vi "ecg_ncs_v7.vi"() -> ()   [LabVIEW 2016]
uses:
  <instrlib>/niUSRP/niUSRP Timestamp.ctl
  C:/Program Files/National Instruments/LabVIEW 2016/examples/Instrument IO/Serial/support/Serial - Settings.ctl
  State.ctl
  <vilib>/Instr/_visa.llb/VISA Configure Serial Port (Instr).vi
  <instrlib>/niUSRP/niUSRP Fetch Rx Data (2D CDB).vi
  <instrlib>/niUSRP/niUSRP Write Tx Data (2D CDB).vi
panel:
  in  "Tab Control 3":enum32{"ECG Sample", "ECG"}(tab)
  out "?":i32(graph)
  out "?":i16(graph)
  in  "maxWrite":i32=2000
  out "size(s) 2":i32
  out "size(s)":i32
  in  "File Name 2":string="Test"
  in  "Path 2":path=path "D:/Research/SummerFall17Spring18/CnC/NCS/EcgNcsCorrelation/Labview Codes/ECG_NCS"
  out "#Loop = #Packets Received":i32
  out "ECGsample":i16
  out "PhNcs":dbl[](array[numeric])
  out "AmpNcs":dbl[](array[numeric])
  out "AmpNcsDS":dbl[](array[numeric])
  out "PhNcsDS":dbl[](array[numeric])
  out "error IO 2":errorcluster={"status"=FALSE, "code"=-1074118647, "source"=""}
  in  "Serial Settings":T1={"baud rate"=57600, "data bits"=8, "parity"=enum."None", "stop bits"=10, "flow control"=0} {"flow control" items=["None"=0, "XON/XOFF"=1, "RTS/CTS"=2, "DTR/DSR"=4]; "stop bits" items=["1.0"=10, "1.5"=15, "2.0"=20]; "data bits" min=5 max=8 step=1; "baud rate" items=["75"=75, "110"=110, "134"=134, "150"=150, "300"=300, "600"=600, "1200"=1200, "1800"=1800, "2400"=2400, "4800"=4800, "7200"=7200, "9600"=9600, "14400"=14400, "19200"=19200, "28800"=28800, "38400"=38400, "56000"=56000, "57600"=57600, "115200"=115200, "128000"=128000, "230400"=230400]}
  in  "VISA resource name":refnum<visa-resource-name>="bmd101"
  in  "byte count":u32=1
  out "Coerced Rx IQ Rate":dbl
  in  "Sampling Rate":i32=500
  out "Gain":dbl=-15.0
  out "Bandwidth":dbl=56000000.0
  out "Coerced Carrier Frequency":dbl=2000000000.0 format="%#.17g"
  out "Coerced Tx IQ rate":dbl=1000000.0
  out "error IO":errorcluster={"status"=FALSE, "code"=-1074118647, "source"=""}
  in  "Rx Number of Samples":i32=10000
  in  "Tab Control 2":enum32{"NI-294x/295x", "NI-2900/2901"}(tab)=enum."NI-2900/2901"
  in  "Rx carrier frequency [Hz]":dbl=2000000000.0 format="%#_6p"
  in  "Tx carrier frequency [Hz]":dbl=1000000000.0 format="%#_6p"
  in  "Start Trigger Time":T2={"whole seconds"=1, "fractional seconds"=0.0}
  in  "Tab Control":T3(tab)
  out "?":dbl(graph)
  out "?":dbl(graph)
  out "NCS tag Amp":dbl[](graph)=[0.011967714738528729, 0.012021355192189592, 0.012015275039596582, 0.011969166030167903, 0.011958890166168242, 0.012007893820858737, 0.012022893722444085, 0.011978222225113794, 0.011969989939463181, 0.012003099640895068]
  out "NCS tag Phase":dbl[](graph)=[0.011967714738528729, 0.012021355192189592, 0.012015275039596582, 0.011969166030167903, 0.011958890166168242, 0.012007893820858737, 0.012022893722444085, 0.011978222225113794, 0.011969989939463181, 0.012003099640895068]
  out "Tag Amp":dbl[](graph)
  out "Tag Phase":dbl[](graph)
  out "Tx Waveform Graph":waveform(dbl)[](graph)
  in  "Stop":bool
  in  "Tone Amplitude":dbl=0.707 step=0.05 format="%#.6g"
  in  "Tone  Frequency":dbl=5000.0 format="%#_6p"
  in  "Tx Waveform Size":dbl=2000.0
  in  "Device Name":refnum<k15>="MyB200"
  in  "Tx Gain":dbl=28.0 format="%#_6f"
  in  "Tx IQ Rate":dbl=1000000.0 format="%#_6p"
  in  "Rx Gain":dbl=32.0 format="%#_6f"
  in  "Rx IQ Rate":dbl=1000000.0 format="%#_6p"
  # "Rx Settings"
  # "Tx Settings"
  # "Note that on the NI-2900 and NI-2901, both Rx channels share an LO and both Tx channels share an LO. However, on the NI-294x/295x devices, Rx and Tx of channel 0 share an LO and Rx and Tx of channel 1 share an LO."
  # "Rx: Number of samples should be 1e6/512 in one loop."
  # "This Tx graph should always have end and start tied up since this is being sent in a loop continuously. Otherwise phase jumps will be noticed."
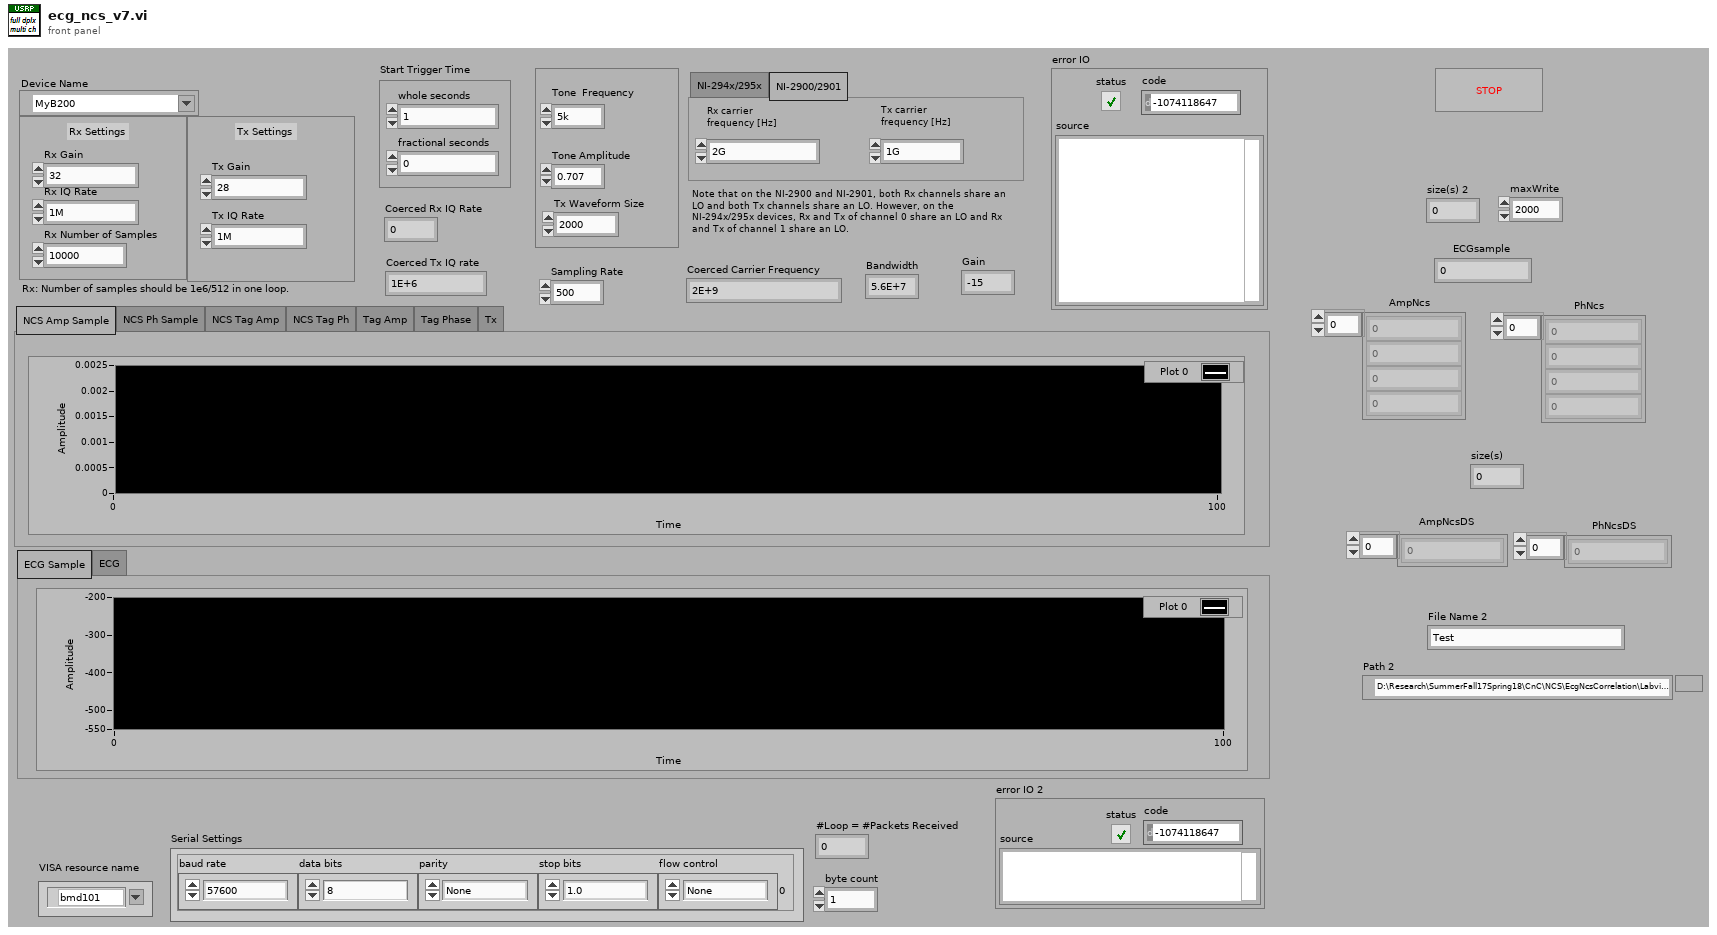
[diagram p1: front panel]
types:
  T1 = typedef "Serial - Settings.ctl" = cluster{"baud rate":u32, "data bits":u16, "parity":enum16{"None", "Odd", "Even", "Mark", "Space"}, "stop bits":u16, "flow control":u16}
  T2 = typedef "niUSRP Timestamp.ctl" = cluster{"whole seconds":u64, "fractional seconds":dbl}
  T3 = enum32{"NCS Amp Sample", "NCS Ph Sample", "NCS Tag Amp", "NCS Tag Ph", "Tag Amp", "Tag Phase", "Tx"}
  T4 = typedef "State.ctl" = enum16{"Initialize", "get byte", "check", "packet received", "packet approved"}
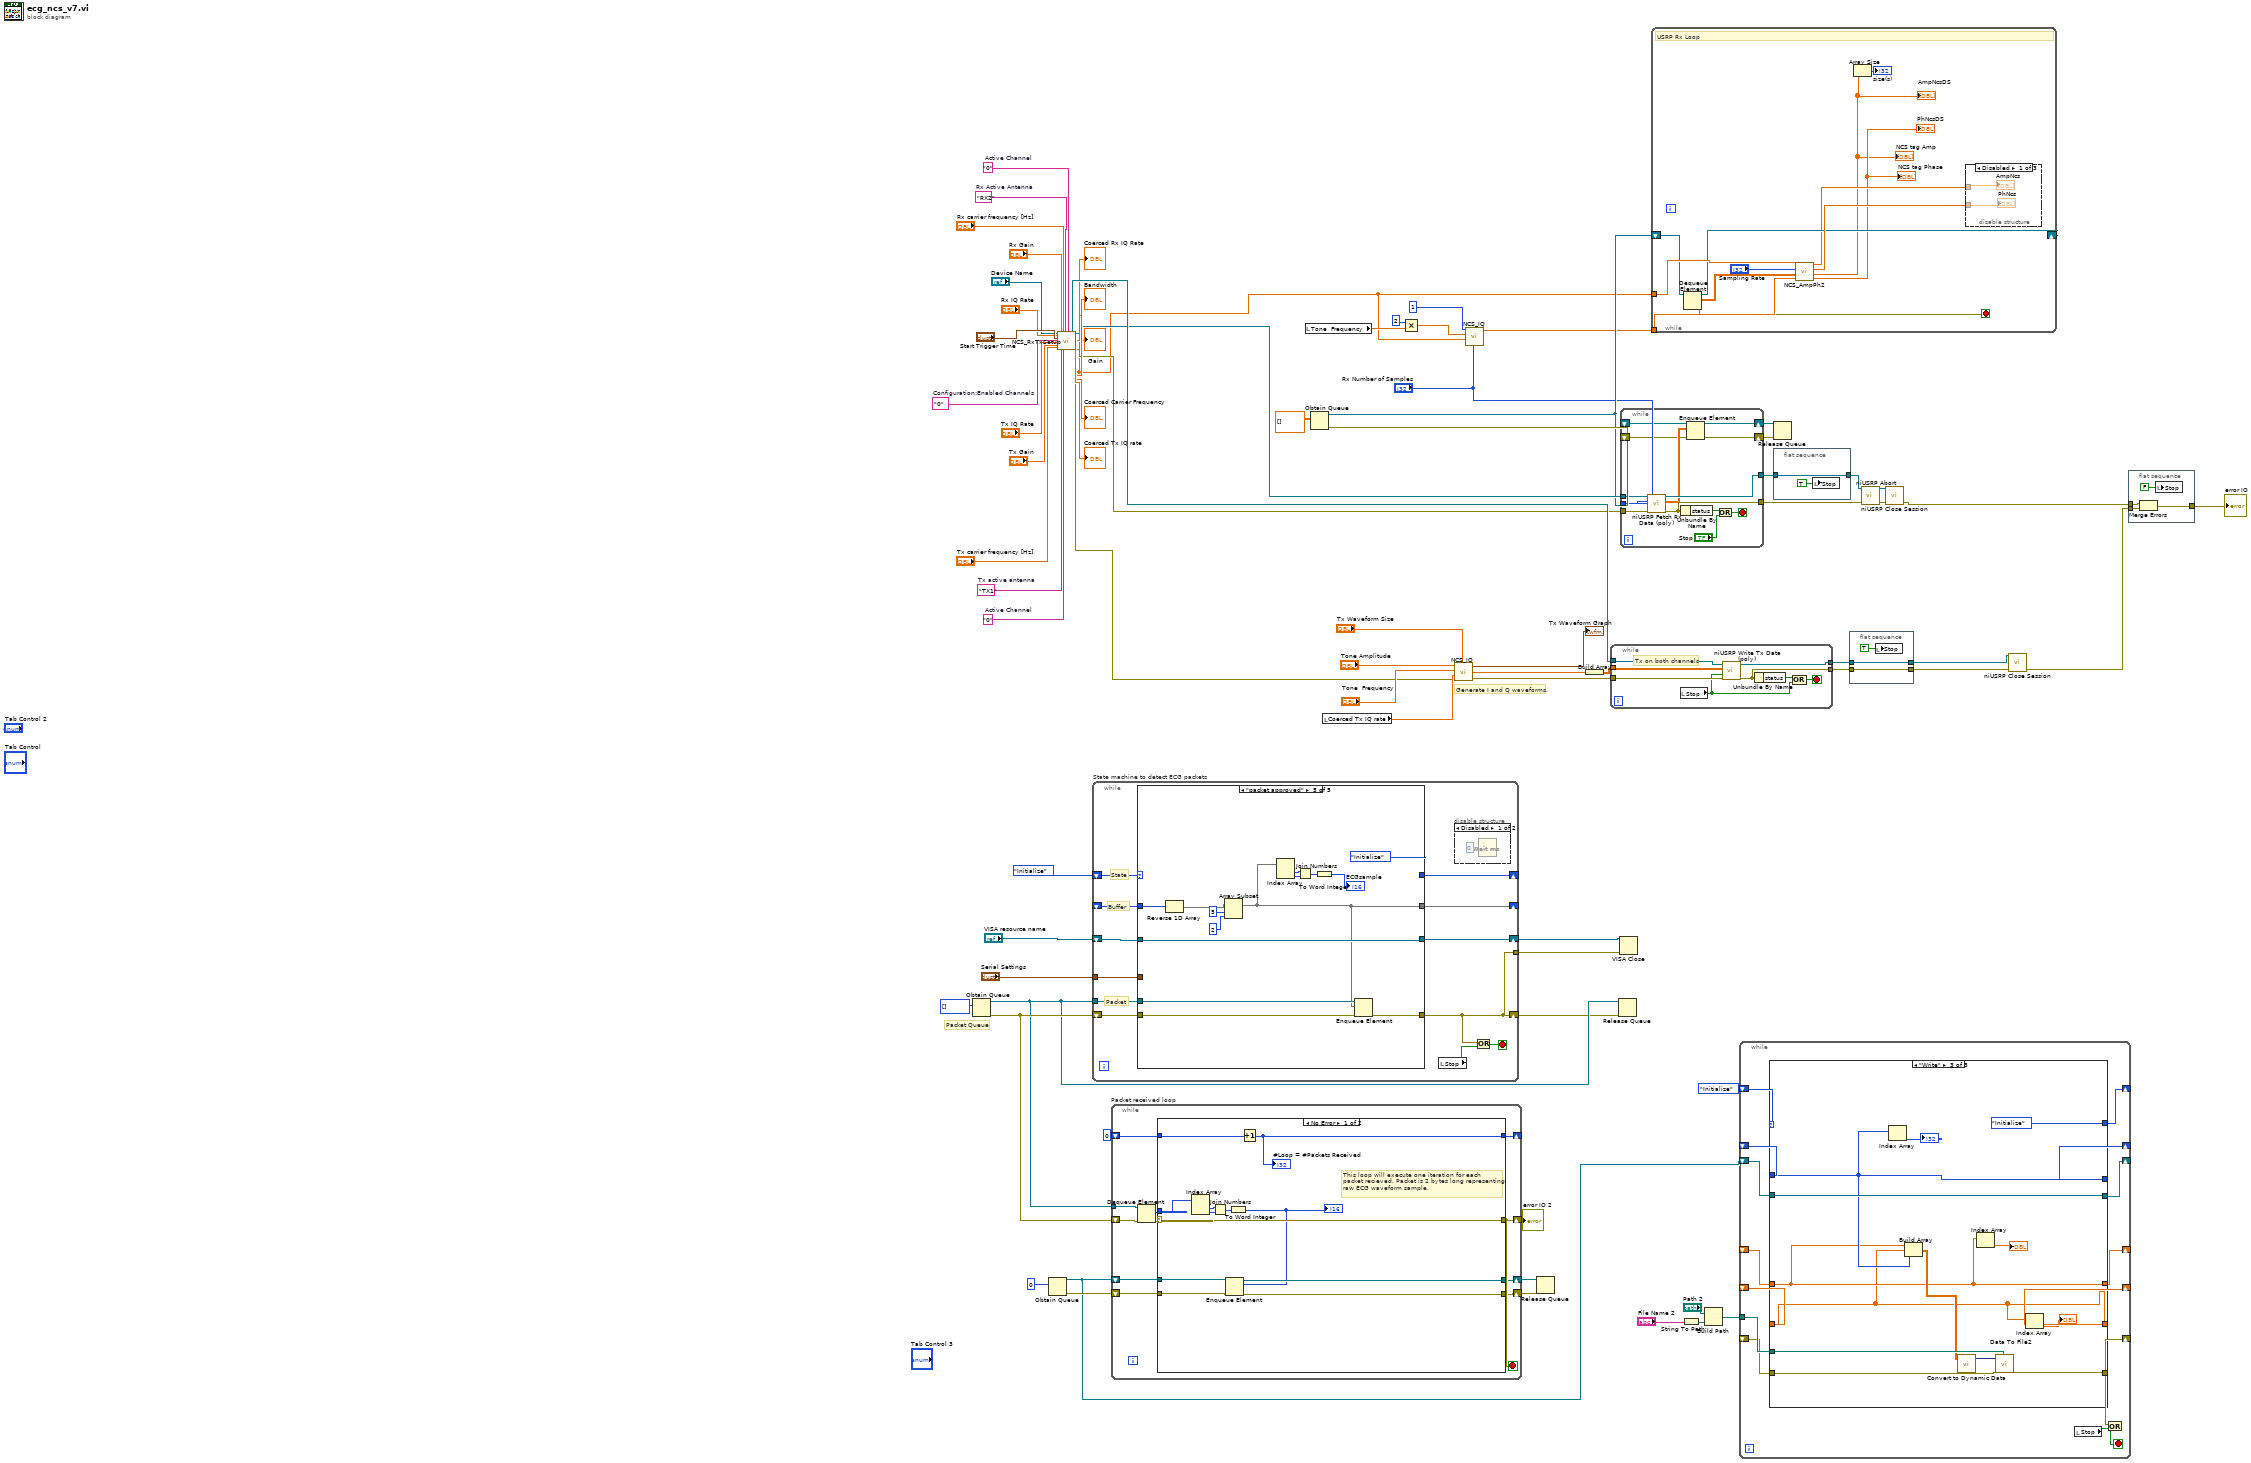
[diagram p0: block diagram]
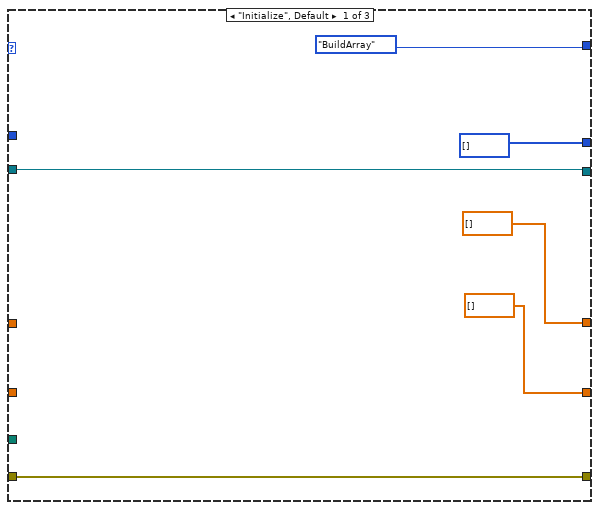
[diagram p2: hidden frame]
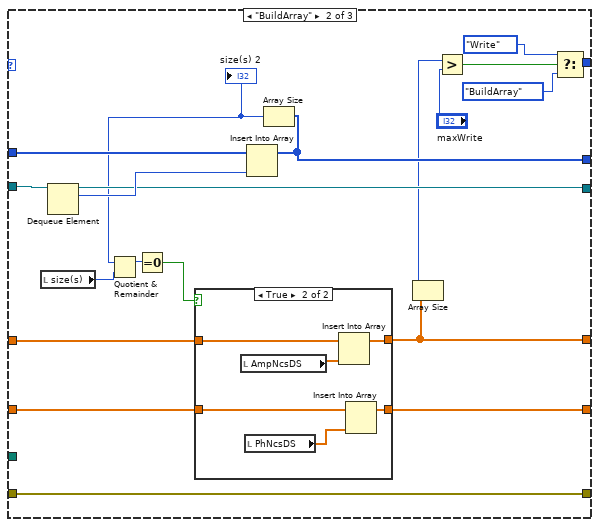
[diagram p3: hidden frame]
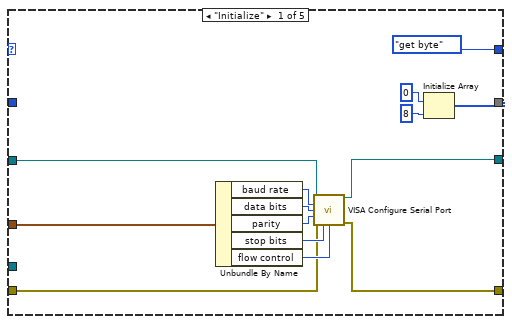
[diagram p7: hidden frame]
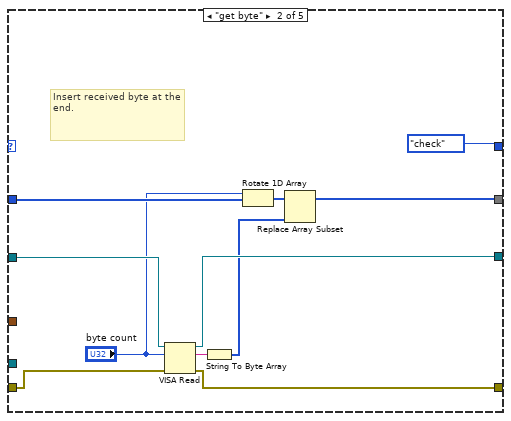
[diagram p8: hidden frame]
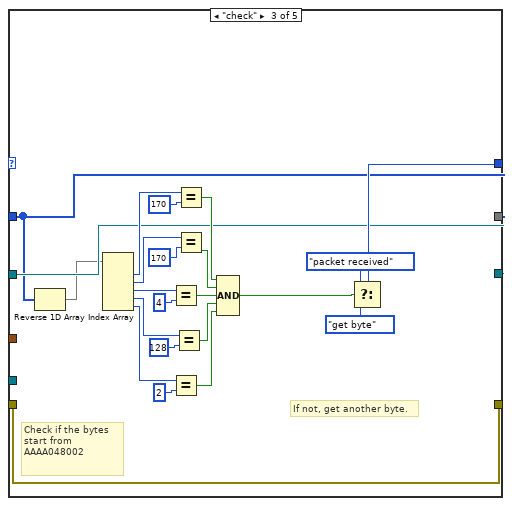
[diagram p9: hidden frame]
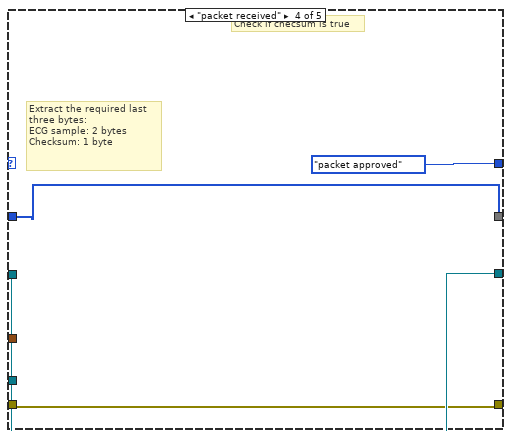
[diagram p10: hidden frame]
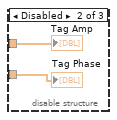
[diagram p11: hidden frame]
diagram:
  w36 = "0"  # Active Channel
  w37 = "0"  # Active Channel
  w66 = "RX2"  # Rx Active Antenna
  w62 = "TX1"  # Tx active antenna
  w51 = "0"  # Configuration:Enabled Channels
  # "Packet Queue"
  # "Generate I and Q waveforms."
  n1 = Obtain Queue(element data type=u8[] []) -> (queue out=w32:refnum<queue>, error out=w33:errorcluster)  [unwired: 4 in, 1 out]
  n2 = Obtain Queue(element data type=0) -> (queue out=w1:refnum<queue>, error out=w4:errorcluster)  [unwired: 4 in, 1 out]
  n3 = call "NCS_RxTxSetup.vi"("IVI Refnum in"="Device Name", "Rx IQ Rate"="Rx IQ Rate", "Start Trigger Time"="Start Trigger Time", "Configuration:Enabled Channels"=w51, "Tx IQ Rate"="Tx IQ Rate", "Tx Gain"="Tx Gain", "Tx carrier frequency [Hz]"="Tx carrier frequency [Hz]", "Rx Gain"="Rx Gain", "Tx active antenna"=w62, "Rx carrier frequency [Hz]"="Rx carrier frequency [Hz]", "Active Channel"=w36, "Rx Active Antenna"=w66, "Active Channel 2"=w37) -> ("session handle out"=w73:refnum<k15>, "IVI Refnum out"=w22:refnum<k15>, "Coerced Rx IQ Rate"=w12:dbl, "Bandwidth"=→"Bandwidth":dbl, "Gain"=→"Gain":dbl, "Carrier Frequency"=→"Coerced Carrier Frequency":dbl, "IQ Rate 2"=→"Coerced Tx IQ rate":dbl, "error out"=w23:errorcluster)  [unwired: 7 in]
  "Coerced Rx IQ Rate" <- w12
  n4 = while "State machine to detect ECG packets" {
    shift-right: [w76] -> w27
    shift-left: w33 -> [w82]
    shift-right: [w85] -> _
    shift-left: State."Initialize" ("State") -> [w84]
    shift-right: [w81] -> _
    shift-left: _ -> [w83]
    tunnel: w32 -> [w80]
    shift-right: [w79] -> w28
    shift-left: "VISA resource name" -> [w78]
    tunnel: "Serial Settings" -> [w77]
    tunnel: [w76] -> w26
    stop <- w75 stop-if-true
    # "State"
    # "Buffer"
    # "Packet"
    n5 = case shown="\"packet approved\"" w84 {
      tunnel: [w97 w109 w113 w136 w140] -> w81
      tunnel: [State."get byte" ("State") State."check" ("f") w133 State."packet approved" ("State") State."Initialize" ("State")] -> w85
      tunnel: w83 -> [_ w102 w113 w136 w145]
      tunnel: w82 -> [w91 w106 w134 w137 w148]
      tunnel: [w90 w105 w134 w137 w147] -> w76
      tunnel: w80 -> [_ _ _ _ w149]
      tunnel: [w89 w107 w114 w138 w146] -> w79
      tunnel: w78 -> [w88 w108 w114 w138 w146]
      tunnel: w77 -> [w87 _ _ _ _]
      frame "Initialize" {
        n6 = Unbundle By Name(w87) -> ("baud rate"=w96:u32, "data bits"=w95:u16, "parity"=w94:enum16{"None", "Odd", "Even", "Mark", "Space"}, "stop bits"=w93:u16, "flow control"=w92:u16)
        n7 = call-poly "VISA Configure Serial Port"("VISA resource name"=w88, "baud rate (9600)"=w96, "data bits (8)"=w95, "parity (0:none)"=w94, "error in (no error)"=w91, "stop bits (10: 1 bit)"=w93, "flow control (0:none)"=w92) -> ("VISA resource name out"=w89:refnum<visa-resource-name>, "error out"=w90:errorcluster)  [unwired: 3 in, 4 out]
        n8 = Initialize Array(u8 0, 8 ("dimension size")) -> (w97:u8[])
      }
      frame "get byte" {
        # "Insert received byte at the end."
        n9 = VISA Read(VISA resource name=w108, byte count="byte count", error in (no error)=w106) -> (VISA resource name out=w107:refnum<visa-resource-name>, read buffer=w104:string, error out=w105:errorcluster)  [unwired: 1 out]
        n10 = String To Byte Array(string=w104) -> (unsigned byte array=w103:u8[])
        n11 = Rotate 1D Array(1:w102, 2:"byte count") -> (0:w110:u8[])
        n12 = Replace Array Subset(array=w110, new element=w103) -> (w109:u8[])  [unwired: 1 in]
      }
      frame "check" {
        # "If not, get another byte."
        # "Check if the bytes start from AAAA048002"
        n13 = Reverse 1D Array(array=w113) -> (reversed array=w112:u8[])
        n14 = Index Array(array=w112) -> (element #1=w120:u8, element #2=w119:u8, element #3=w118:u8, element #4=w117:u8, element #5=w116:u8)  [unwired: 5 in]
        n15 = Equal?(x=w118, y=u8 4 ("element")) -> (x = y?=w123:bool)
        n16 = Equal?(x=w116, y=u8 2 ("element")) -> (x = y?=w121:bool)
        n17 = Equal?(x=w117, y=u8 128 ("element")) -> (x = y?=w122:bool)
        n18 = Equal?(x=w120, y=u8 170 ("element")) -> (x = y?=w125:bool)
        n19 = Equal?(x=w119, y=u8 170 ("element")) -> (x = y?=w124:bool)
        n20 = Compound Arithmetic op=AND(w125, w124, w123, w122, w121) -> (w115:bool)
        n21 = Select(t=State."packet received" ("f"), s=w115, f=State."get byte") -> (s? t:f=w133:T4)
      }
      frame "packet received" {
        # "Check if checsum is true"
        # "Extract the required last three bytes: \nECG sample: 2 bytes\nChecksum: 1 byte"
      }
      frame "packet approved" {
        n22 = Reverse 1D Array(array=w145) -> (reversed array=w144:u8[])
        n23 = Array Subset(array=w144, index=5, length=2 ("index")) -> (w140:u8[])
        n24 = Index Array(array=w140) -> (element #1=w143:u8, element #2=w142:u8)  [unwired: 2 in]
        n25 = Join Numbers(hi=w143, lo=w142) -> ((hi.lo)=w141:u16)
        n26 = To Word Integer(number=w141) -> (16bit integer=→"ECGsample":i16)
        n27 = Enqueue Element(queue=w149, element=w140, error in (no error)=w148) -> (error out=w147:errorcluster)  [unwired: 1 in, 2 out]
      }
    }
    n28 = local read "Stop"() -> (w74:bool)
    n29 = disable-structure shown="Disabled" {
      frame Disabled {
        n30 = Wait (ms)(milliseconds to wait=u32 0) -> ()  [unwired: 1 out]
      }
      frame Enabled {
      }
    }
    n31 = Or(x=w76, y=w74) -> (x .or. y?=w75:bool)
  }
  n32 = while "Packet received loop" {
    shift-right: [w159] -> w29
    shift-left: w33 -> [w163]
    tunnel: w32 -> [w162]
    shift-right: [w157] -> _
    shift-left: 0 -> [w158]
    shift-right: [w154] -> w2
    shift-left: w1 -> [w156]
    shift-right: [w153] -> w3
    shift-left: w4 -> [w155]
    stop <- w159 stop-if-true
    n33 = Dequeue Element(queue=w162, error in (no error)=w163) -> (element=w161:u8[], error out=w160:errorcluster)  [unwired: 1 in, 2 out]
    n34 = case shown="No Error" w160 {
      selector: w160 -> [w169 w179]
      tunnel: w161 -> [w175 _]
      tunnel: [w169 w179] -> w159
      tunnel: w158 -> [w171 w178]
      tunnel: [w170 w178] -> w157
      tunnel: w156 -> [w168 w177]
      tunnel: w155 -> [w167 w176]
      tunnel: [w166 w177] -> w154
      tunnel: [w165 w176] -> w153
      frame No Error {
        # "This loop will execute one iteration for each\npacket recieved. Packet is 2 bytes long representing \nraw ECG waveform sample."
        n35 = Index Array(array=w175) -> (element #1=w174:u8, element #2=w173:u8)  [unwired: 2 in]
        n36 = Join Numbers(hi=w174, lo=w173) -> ((hi.lo)=w172:u16)
        n37 = To Word Integer(number=w172) -> (16bit integer=w164:i16)
        "?" <- w164
        n38 = Enqueue Element(queue=w168, element=w164, error in (no error)=w167) -> (queue out=w166:refnum<queue>, error out=w165:errorcluster)  [unwired: 1 in, 1 out]
        n39 = Increment(x=w171) -> (x+1=w170:i32)
        "#Loop = #Packets Received" <- w170
      }
      frame Error {
      }
    }
  }
  "error IO 2" <- w29
  n40 = local read "Tone  Frequency"() -> (w50:dbl)
  n41 = Obtain Queue(element data type=dbl[][] []) -> (queue out=w16:refnum<queue>, error out=w19:errorcluster)  [unwired: 4 in, 1 out]
  n42 = local read "Coerced Tx IQ rate"() -> (w46:dbl)
  n43 = Multiply(x=2, y=w50) -> (x*y=w13:dbl)
  n44 = call "NCS_IQ.vi"("Tone Amplitude"="Tone Amplitude", "Waveform Size"="Tx Waveform Size", "Tone Frequency"="Tone  Frequency", "Coerced IQ rate"=w46, "error in (no error)"=w23) -> ("IQ waveform"=→"Tx Waveform Graph":waveform(dbl)[], "IQ waveform array"=w44:cdb[], "error out"=w45:errorcluster)  [unwired: 1 in]
  n45 = call "NCS_IQ.vi"("Tone Amplitude"=1, "Waveform Size"="Rx Number of Samples", "Tone Frequency"=w13, "Coerced IQ rate"=w12) -> ("IQ waveform array"=w15:cdb[])  [unwired: 2 in, 2 out]
  n46 = Release Queue(queue=w2, error in (no error)=w3) -> ()  [unwired: 1 in, 3 out]
  n47 = Build Array(w44) -> (w70:cdb[][])
  n48 = while {
    tunnel: w73 -> [w187]
    tunnel: w45 -> [w186]
    tunnel: [w184] -> w61
    tunnel: [w182] -> w57
    tunnel: w70 -> [w180]
    stop <- w183 stop-if-true
    # "Tx on both channels"
    n49 = local read "Stop"() -> (w181:bool)
    n50 = call-poly <instrlib>:"niUSRP Write Tx Data (poly).vi"("session handle"=w187, "data"=w180, "end of data?"=w181, "error in (no error)"=w186) -> ("session handle out"=w182:refnum<k15>, "error out"=w184:errorcluster)  [unwired: 10 in]
    n51 = Unbundle By Name(w184) -> ("status"=w185:bool)
    n52 = Compound Arithmetic op=OR(w185, w181) -> (w183:bool)
  }
  n53 = Release Queue(queue=w32, error in (no error)=w27) -> ()  [unwired: 1 in, 3 out]
  n54 = VISA Close(VISA resource name=w28, error in (no error)=w26) -> ()  [unwired: 1 out]
  n55 = while {
    tunnel: w23 -> [w200]
    tunnel: w22 -> [w199]
    tunnel: [w198] -> w21
    tunnel: [w190] -> w20
    shift-right: [w194] -> w18
    shift-left: w19 -> [w195]
    shift-right: [w193] -> w17
    shift-left: w16 -> [w197]
    tunnel: "Rx Number of Samples" -> [w192]
    stop <- w189 stop-if-true
    n56 = call-poly <instrlib>:"niUSRP Fetch Rx Data (poly).vi"("session handle"=w199, "number of samples"=w192, "error in (no error)"=w200) -> ("session handle out"=w198:refnum<k15>, "data"=w196:cdb[][], "error out"=w190:errorcluster)  [unwired: 9 in, 1 out]
    n57 = Unbundle By Name(w190) -> ("status"=w191:bool)
    n58 = Enqueue Element(queue=w197, element=w196, error in (no error)=w195) -> (queue out=w193:refnum<queue>, error out=w194:errorcluster)  [unwired: 1 in, 1 out]
    n59 = Or(x=w191, y="Stop") -> (x .or. y?=w189:bool)
  }
  n60 = while {
    tunnel: w12 -> [w212]
    shift-right: [w208] -> _
    shift-left: w16 -> [w209]
    tunnel: w15 -> [w206]
    stop <- w205 stop-if-true
    # "USRP Rx Loop"
    n61 = Dequeue Element(queue=w209) -> (queue out=w208:refnum<queue>, element=w207:dbl[][], error out=w205:errorcluster)  [unwired: 2 in, 1 out]
    n62 = call "NCS_AmpPh2.vi"("IQ"=w206, "data"=w207, "Sampling Rate"="Sampling Rate", "Coerced Rx IQ Rate"=w212) -> ("Phase DownSampled"=→"NCS tag Phase" →"PhNcsDS":dbl[], "Amp DownSampled"=w201:dbl[], "Phase"=w210:dbl[], "Amplitude"=w204:dbl[])  [unwired: 3 in, 1 out]
    "NCS tag Amp" <- w201
    "AmpNcsDS" <- w201
    n63 = Array Size(array=w201) -> (size(s)=→"size(s)":i32)
    n64 = disable-structure shown="Disabled" {
      disable-tunnel: w204 -> [w213 w216 _]
      disable-tunnel: w210 -> [w214 w215 _]
      frame Disabled {
        "AmpNcs" <- w213
        "PhNcs" <- w214
      }
      frame Disabled {
        "Tag Amp" <- w216
        "Tag Phase" <- w215
      }
      frame Enabled {
      }
    }
  }
  n65 = String To Path(string="File Name 2") -> (path=w10:path)
  n66 = Build Path(base path="Path 2", name or relative path=w10) -> (appended path=w6:path)
  n67 = while {
    shift-right: [w230] -> _
    shift-left: _ -> [w231]
    shift-right: [w228] -> _
    shift-left: _ -> [w229]
    shift-right: [w226] -> _
    shift-left: enum16{"Initialize", "BuildArray", "Write"}."Initialize" -> [w227]
    tunnel: w6 -> [w225]
    shift-right: [w222] -> _
    shift-left: _ -> [w221]
    shift-right: [w219] -> _
    shift-left: w1 -> [w220]
    shift-right: [w218] -> _
    shift-left: _ -> [w217]
    stop <- w223 stop-if-true
    n68 = case shown="\"Write\"" w227 {
      tunnel: w231 -> [_ w257 w271]
      tunnel: [i32[] [] w255 w271] -> w230
      tunnel: w229 -> [_ w256 w267]
      tunnel: [dbl[] [] w244 w267] -> w228
      tunnel: [enum16{"Initialize", "BuildArray", "Write"}."BuildArray" w250 enum16{"Initialize", "BuildArray", "Write"}."Initialize"] -> w226
      tunnel: w225 -> [_ _ w276]
      tunnel: [w236 w249 w274] -> w222
      tunnel: w221 -> [w236 w249 w273]
      tunnel: w220 -> [w235 w247 w272]
      tunnel: [w235 w246 w272] -> w219
      tunnel: [dbl[] [] w239 w269] -> w218
      tunnel: w217 -> [_ w245 w269]
      frame "Initialize", Default {
      }
      frame "BuildArray" {
        n69 = local read "size(s)"() -> (w242:i32)
        n70 = Dequeue Element(queue=w247) -> (queue out=w246:refnum<queue>, element=w248:i32)  [unwired: 2 in, 2 out]
        n71 = Insert Into Array(array=w257, new element=w248) -> (w255:i32[])  [unwired: 1 in]
        n72 = Array Size(array=w255) -> (size(s)=w243:i32)
        "size(s) 2" <- w243
        n73 = Quotient & Remainder(x=w243, y=w242) -> (x-y*floor(x/y)=w241:i32)  [unwired: 1 out]
        n74 = Equal To 0?(x=w241) -> (x = 0?=w240:bool)
        n75 = case shown="True" w240 {
          tunnel: w256 -> [w258 w261]
          tunnel: [w258 w260] -> w244
          tunnel: w245 -> [w259 w263]
          tunnel: [w259 w262] -> w239
          frame False {
          }
          frame True {
            n76 = local read "AmpNcsDS"() -> (w265:dbl[])
            n77 = local read "PhNcsDS"() -> (w264:dbl[])
            n78 = Insert Into Array(array=w263, new element=w265) -> (w262:dbl[])  [unwired: 1 in]
            n79 = Insert Into Array(array=w261, new element=w264) -> (w260:dbl[])  [unwired: 1 in]
          }
        }
        n80 = Array Size(array=w239) -> (size(s)=w238:i32)
        n81 = Greater?(x=w238, y="maxWrite") -> (0:w253:bool)
        n82 = Select(t=enum16{"Initialize", "BuildArray", "Write"}."Write", s=w253, f=enum16{"Initialize", "BuildArray", "Write"}."BuildArray") -> (s? t:f=w250:enum16{"Initialize", "BuildArray", "Write"})
      }
      frame "Write" {
        n83 = Index Array(array=w271) -> (element=→"?":i32)  [unwired: 1 in]
        n84 = Build Array(w269, w267, w271) -> (w275:dbl[][])
        n85 = call "Convert to Dynamic Data"("2D Array"=w275) -> ("Dynamic Data Type"=w277:dynamicdata)  [unwired: 3 in]
        n86 = Index Array(array=w269) -> (element=→"?":dbl)  [unwired: 1 in]
        n87 = call "Data To File2"("Signals"=w277, "error in (no error)"=w273, "Filename"=w276) -> ("error out"=w274:errorcluster)  [unwired: 14 in, 2 out]
        n88 = Index Array(array=w267) -> (element=→"?":dbl)  [unwired: 1 in]
      }
    }
    n89 = local read "Stop"() -> (w224:bool)
    n90 = Or(x=w222, y=w224) -> (x .or. y?=w223:bool)
  }
  n91 = Release Queue(queue=w17, error in (no error)=w18) -> ()  [unwired: 1 in, 3 out]
  n92 = flat-sequence {
    tunnel: [w279] -> w59
    tunnel: w21 -> [w279]
    frame #0 {
      n93 = local write "Stop"(TRUE ("STOP")) -> ()
    }
  }
  n94 = flat-sequence {
    tunnel: [w282] -> w60
    tunnel: w61 -> [w282]
    tunnel: [w281] -> w58
    tunnel: w57 -> [w281]
    frame #0 {
      n95 = local write "Stop"(TRUE ("STOP")) -> ()
    }
  }
  n96 = call <instrlib>:"niUSRP Abort.vi"("session handle"=w59, "error in (no error)"=w20) -> ("session handle out"=w72:refnum<k15>, "error out"=w71:errorcluster)  [unwired: 12 in]
  n97 = call <instrlib>:"niUSRP Close Session.vi"("session handle"=w72, "error in (no error)"=w71) -> ("error out"=w54:errorcluster)  [unwired: 13 in]
  n98 = call <instrlib>:"niUSRP Close Session.vi"("session handle"=w58, "error in (no error)"=w60) -> ("error out"=w56:errorcluster)  [unwired: 13 in]
  n99 = flat-sequence {
    tunnel: w56 -> [w286]
    tunnel: [w285] -> w55
    tunnel: w54 -> [w284]
    frame #0 {
      n100 = Merge Errors(w284, w286) -> (w285:errorcluster)
      n101 = local write "Stop"(FALSE ("STOP")) -> ()
    }
  }
  "error IO" <- w55
